vi "836Elevator_Encoder.vi"(2 "Elevator Encoder Ref":string="Elevator Encoder") -> (0 "Output":dbl)   [LabVIEW 2011]
uses:
  Robot Global Data.vi
panel:
  out "Code Output":dbl(graph)
  in  "Zero Encoder":dbl(slide)=-0.050505050505050594 scale=-5.0..5.0
  out "Offset":dbl
  out "Last":dbl(knob) scale=0.0..4.98
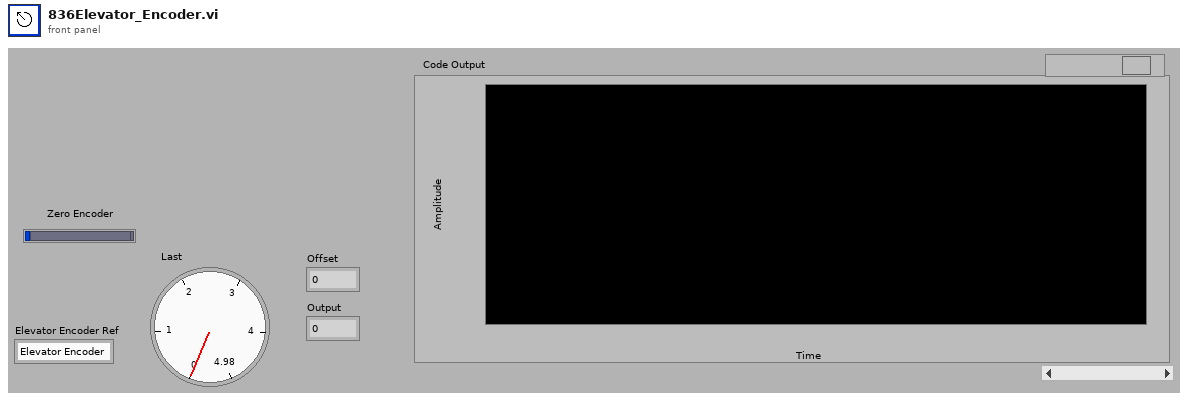
[diagram p1: front panel]
types:
  T1 = typedef "WPI_AnalogChannelDevRef.ctl" = cluster{"DevStatus":errorcluster, "Analog Module":T2, "Analog Channel":T3}
  T2 = typedef "FPGA_TypedefAnalogModule.ctl" = enum16{"Analog Module 1", "Analog Module 2"}
  T3 = typedef "FPGA_AIChannel.ctl" = enum8{"AI 1", "AI 2", "AI 3", "AI 4", "AI 5", "AI 6", "AI 7", "AI 8", "Invalid"}
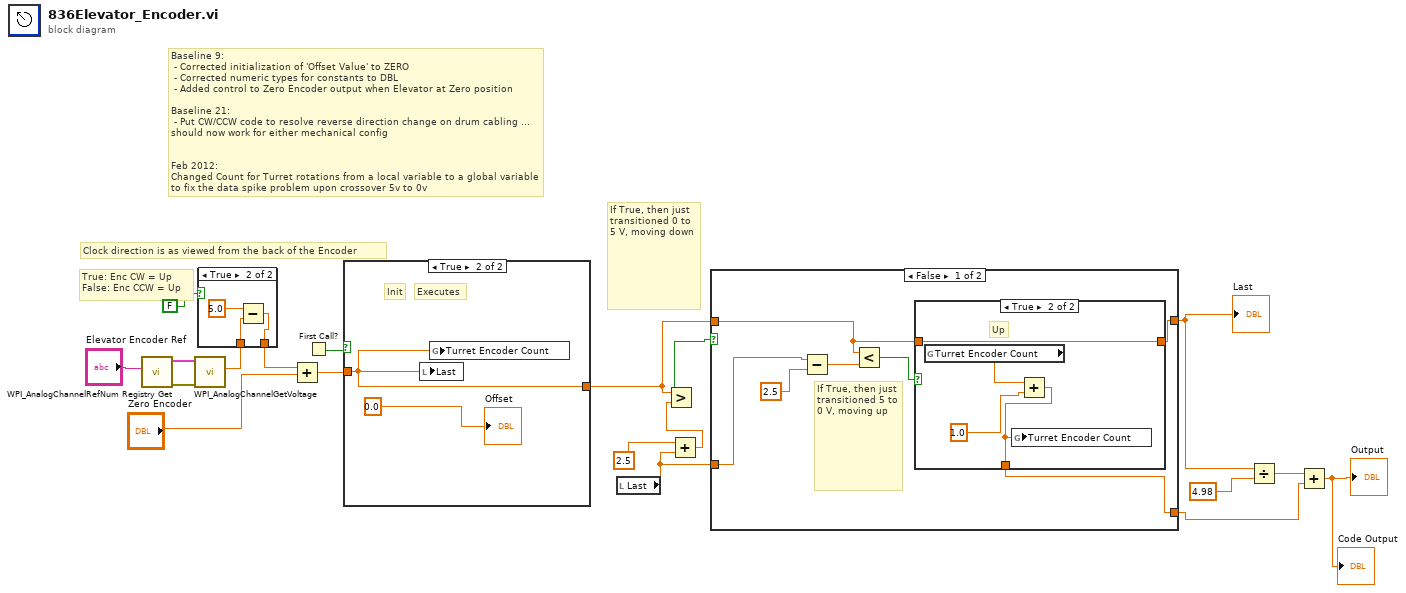
[diagram p0: block diagram]
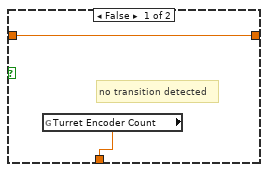
[diagram p3: hidden frame]
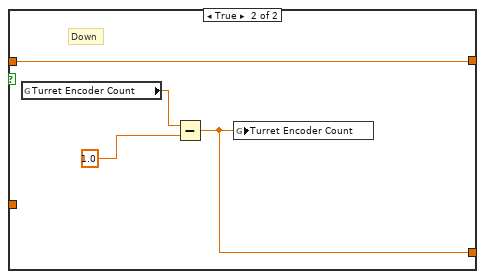
[diagram p4: hidden frame]
diagram:
  # "Clock direction is as viewed from the back of the Encoder"
  # "True: Enc CW = Up\nFalse: Enc CCW = Up"
  # "Baseline 9:\n - Corrected initialization of 'Offset Value' to ZERO\n - Corrected numeric types for constants to DBL\n - Added control to Zero Encoder output when Elevator at Zero position\n\nBaseline 21:\n - Put CW/CCW code to resolve reverse direction change on drum cabling ... should now work for either mechanical config\n \n\nFeb 2012:\nChanged Count for Turret rotations from a local variable to a global variable to fix the data spike problem upon crossover 5v to 0v"
  # "If True, then just transitioned 0 to 5 V, moving down"
  n1 = call <vilib>:"WPI_AnalogChannelRefNum Registry Get.vi"("refnum name"="Elevator Encoder Ref") -> ("error out"=w10:errorcluster, "AIDeviceRef"=w11:T1)  [unwired: 1 in, 8 out]
  n2 = call <vilib>:"WPI_AnalogChannelGetVoltage.vi"("error in (no error)"=w10, "AIDeviceRef"=w11) -> ("Voltage"=w5:dbl)  [unwired: 9 out]
  n3 = case shown="True" FALSE {
    tunnel: w5 -> [w20 w22]
    tunnel: [w20 w21] -> w4
    frame False {
    }
    frame True {
      n4 = Subtract(x=5.0, y=w22) -> (x-y=w21:dbl)
    }
  }
  n5 = Add(x=w4, y="Zero Encoder") -> (x+y=w3:dbl)
  n6 = First Call?() -> (First Call?: T/F=w8:bool)
  n7 = case shown="True" w8 {
    tunnel: w3 -> [w24 w25]
    tunnel: [w24 w25] -> w15
    frame False {
    }
    frame True {
      # "Executes"
      # "Init"
      n8 = local write "Last"(w25) -> ()
      n9 = global write "Robot Global Data.vi" "Turret Encoder Count"(w25) -> ()
      "Offset" <- 0.0
    }
  }
  n10 = local read "Last"() -> (w16:dbl)
  n11 = Add(x=2.5, y=w16) -> (x+y=w18:dbl)
  n12 = Greater?(x=w15, y=w18) -> (0:w17:bool)
  n13 = case shown="False" w17 {
    tunnel: w16 -> [w30 _]
    tunnel: w15 -> [w29 w42]
    tunnel: [w28 w42] -> w12
    tunnel: [w27 w40] -> w1
    frame False {
      # "If True, then just transitioned 5 to 0 V, moving up"
      n14 = Subtract(x=w30, y=2.5 ("x")) -> (x-y=w32:dbl)
      n15 = Less?(x=w29, y=w32) -> (x < y?=w31:bool)
      n16 = case shown="True" w31 {
        tunnel: [w35 w39] -> w28
        tunnel: w29 -> [w35 w39]
        tunnel: [w34 w36] -> w27
        frame False {
          # "no transition detected"
          n17 = global read "Robot Global Data.vi" "Turret Encoder Count"() -> (w34:dbl)
        }
        frame True {
          # "Up"
          n18 = global read "Robot Global Data.vi" "Turret Encoder Count"() -> (w37:dbl)
          n19 = Add(x=w37, y=1.0) -> (x+y=w36:dbl)
          n20 = global write "Robot Global Data.vi" "Turret Encoder Count"(w36) -> ()
        }
      }
    }
    frame True {
      # "Down"
      n21 = global read "Robot Global Data.vi" "Turret Encoder Count"() -> (w41:dbl)
      n22 = Subtract(x=w41, y=1.0) -> (x-y=w40:dbl)
      n23 = global write "Robot Global Data.vi" "Turret Encoder Count"(w40) -> ()
    }
  }
  "Last" <- w12
  n24 = Divide(x=w12, y=4.98) -> (x/y=w14:dbl)
  n25 = Add(x=w14, y=w1) -> (x+y=→"Output" →"Code Output":dbl)
